vi "SWERVE_TRAJECTORY_BEGIN.vi"(7 "Starting ChassisSpeeds":T1 {"vOmega" format="%10.3f"; "vY" format="%10.3f"; "vX" format="%10.3f"}, 8 "ABS Odo Initialize":bool, 9 "gyroAngle":T3={"VALUE"=0.0, "COS"=1.0, "SIN"=0.0} {"SIN" format="%13.4f"; "COS" format="%13.4f"; "VALUE" format="%13.4f"}, 10 "Module Positions":T2[](array[typedef]) {"Angle"."SIN" format="%13.4f"; "Angle"."COS" format="%13.4f"; "Angle"."VALUE" format="%13.4f"}, 11 "Trajectory File Name":string="/home/lvuser/natinst/bin/LabVIEW Data/Path 1- segm 1.wpilib.csv") -> ()   [LabVIEW 2023]
uses:
  <vilib>/Rock Robotics/WPI/ThirdParty/JAS_Junk/TrajLib/TypeDef/ROTATION2D.ctl
  <vilib>/Rock Robotics/WPI/ThirdParty/JAS_Junk/TrajLib/TypeDef/SWERVE_DRIVE_MODULE_POSITION.ctl
  <vilib>/Rock Robotics/WPI/ThirdParty/JAS_Junk/TrajLib/SwerveOdometry_New.vi
  <vilib>/Rock Robotics/WPI/ThirdParty/JAS_Junk/TrajLib/Pose2d_New.vi
  <vilib>/Rock Robotics/WPI/ThirdParty/JAS_Junk/TrajLib/Pose2d_getRotation.vi
  <vilib>/Rock Robotics/WPI/ThirdParty/JAS_Junk/TrajLib/Rotation2d_Minus.vi
  <vilib>/Rock Robotics/SystemInterfaces/NetworkCommunication/NetComm_UsageReport_report.vi
  <vilib>/Rock Robotics/WPI/ThirdParty/JAS_Junk/TrajLib/Rotation2d_CreateAngle.vi
  <vilib>/Rock Robotics/WPI/ThirdParty/JAS_Junk/TrajLib/Translation2d_Create.vi
  <vilib>/Rock Robotics/WPI/ThirdParty/JAS_Junk/TrajLib/Rotation2d_UnaryMinus.vi
  <vilib>/Rock Robotics/WPI/ThirdParty/JAS_Junk/TrajLib/Rotation2d_RotateBy.vi
  <vilib>/Rock Robotics/WPI/ThirdParty/JAS_Junk/TrajLib/Rotation2d_CreateXY.vi
  <vilib>/Rock Robotics/WPI/ThirdParty/JAS_Junk/TrajLib/Util_CalcDist.vi
  SWERVE_TRAJECTORY_GLOBALS.vi
  <vilib>/Rock Robotics/WPI/ThirdParty/JAS_Junk/TrajLib/Globals/Util_LibraryGlobals.vi
  <vilib>/Rock Robotics/WPI/ThirdParty/JAS_Junk/TrajLib/Trajectory_Library.lvlib
  <vilib>/Rock Robotics/WPI/ThirdParty/JAS_Junk/TrajLib/TypeDef/CHASSIS_SPEEDS.ctl
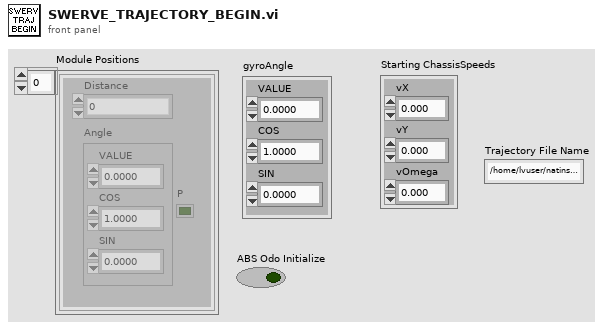
[diagram p1: front panel]
types:
  T1 = typedef "Trajectory_Library.lvlib/CHASSIS_SPEEDS.ctl" = cluster{"vX":dbl, "vY":dbl, "vOmega":dbl}
  T2 = typedef "Trajectory_Library.lvlib/SWERVE_DRIVE_MODULE_POSITION.ctl" = cluster{"Distance":dbl, "Angle":T3, "P":bool}
  T3 = typedef "Trajectory_Library.lvlib/ROTATION2D.ctl" = cluster{"VALUE":dbl, "COS":dbl, "SIN":dbl}
  T4 = typedef "Trajectory_Library.lvlib/SWERVE_DRIVE_ODOMETRY.ctl" = cluster{"POSE":T5, "GyroOffset":T3, "PreviousAngle":T3, "PrevModulePositions":T2[], "NumModules":i32}
  T5 = typedef "Trajectory_Library.lvlib/POSE2D.ctl" = cluster{"TRANSLATION":T6, "ROTATION":T3}
  T6 = typedef "Trajectory_Library.lvlib/TRANSLATION2D.ctl" = cluster{"X":dbl, "Y":dbl}
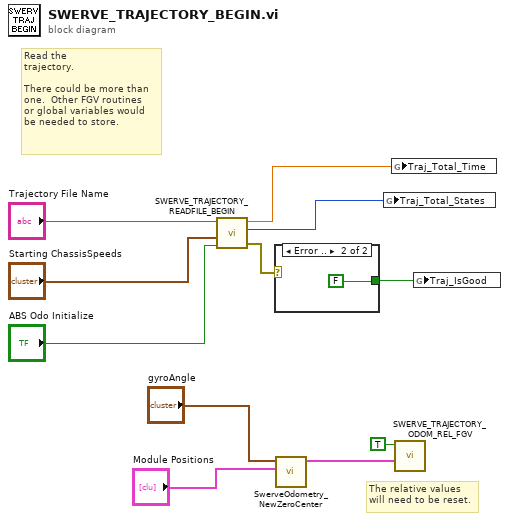
[diagram p0: block diagram]
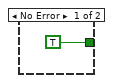
[diagram p2: hidden frame]
diagram:
  # "The relative values\nwill need to be reset."
  # "Read the\ntrajectory.\n\nThere could be more than\none.  Other FGV routines\nor global variables would\nbe needed to store."
  n1 = call "SWERVE_TRAJECTORY_READFILE_BEGIN.vi"("ABS Odo Initialize"="ABS Odo Initialize", "Starting ChassisSpeeds"="Starting ChassisSpeeds", "Trajectory File Name"="Trajectory File Name") -> ("error out"=w11:errorcluster, "Trajectory Items"=w5:i32, "TotalTImeSecs"=w6:dbl)  [unwired: 6 in]
  n2 = case shown="Error .." w11 {
    tunnel: [TRUE FALSE] -> w4
    frame No Error {
    }
    frame Error {
    }
  }
  n3 = call <vilib>:"SwerveOdometry_NewZeroCenter.vi"("Module Positions"="Module Positions", "gyroAngle"="gyroAngle") -> ("SWERVE_DRIVE_ODOMETRY"=w10:T4)  [unwired: 9 in]
  n4 = global write "SWERVE_TRAJECTORY_GLOBALS.vi" "Traj_Total_States"(w5) -> ()
  n5 = global write "SWERVE_TRAJECTORY_GLOBALS.vi" "Traj_Total_Time"(w6) -> ()
  n6 = call "SWERVE_TRAJECTORY_ODOM_REL_FGV.vi"("in SWERVE_DRIVE_ODOMETRY"=w10, "WRITE"=TRUE) -> ()  [unwired: 9 in, 1 out]
  n7 = global write "SWERVE_TRAJECTORY_GLOBALS.vi" "Traj_IsGood"(w4) -> ()
